vi "Power Accuracy Plot Measurement.vi"(4 "Calculated Values":refnum<vi>, 5 "Tolerance (dBm)":cluster{i32[], dbl[]}, 6 "Reset Plot? (F)":bool, 7 "Plots":T2, 8 "error in (no error)":errorcluster, 11 "Measurement Data":T1) -> (0 "error out":errorcluster)   [LabVIEW 2011]
uses:
  TypeDefs/Power Accuracy Measurement Data.ctl
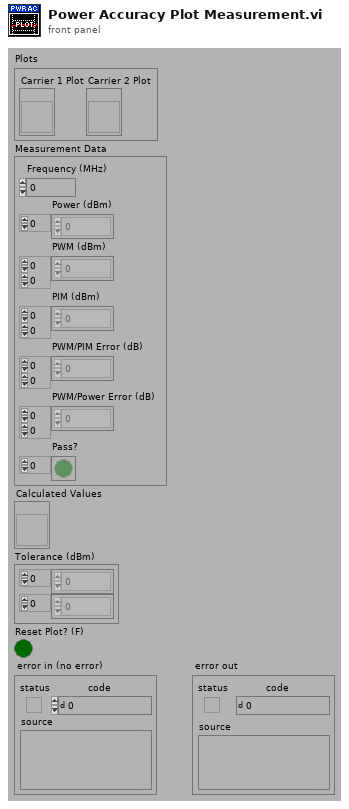
[diagram p1: front panel]
types:
  T1 = typedef "Power Accuracy Measurement Data.ctl" = cluster{"Frequency (MHz)":dbl, "Power (dBm)":i32[], "PWM (dBm)":dbl[][], "PIM (dBm)":dbl[][], "PWM/PIM Error (dB)":dbl[][], "PWM/Power Error (dB)":dbl[][], "Pass?":bool[]}
  T2 = cluster{"Carrier 1 Plot":refnum<vi>, "Carrier 2 Plot":refnum<vi>}
  T3 = cluster{"Array Constant":dbl[], "Array Constant":dbl[]}[]
  T4 = cluster{"Power (dBm)":i32[], "PWM/Power Error (dB)":dbl[]}
  T5 = cluster{"Power (dBm)":i32[], "PWM/PIM Error (dB)":dbl[]}
  T6 = cluster{"Power (dBm)":i32[], "PWM/Power Error (dB)":dbl[]}[]
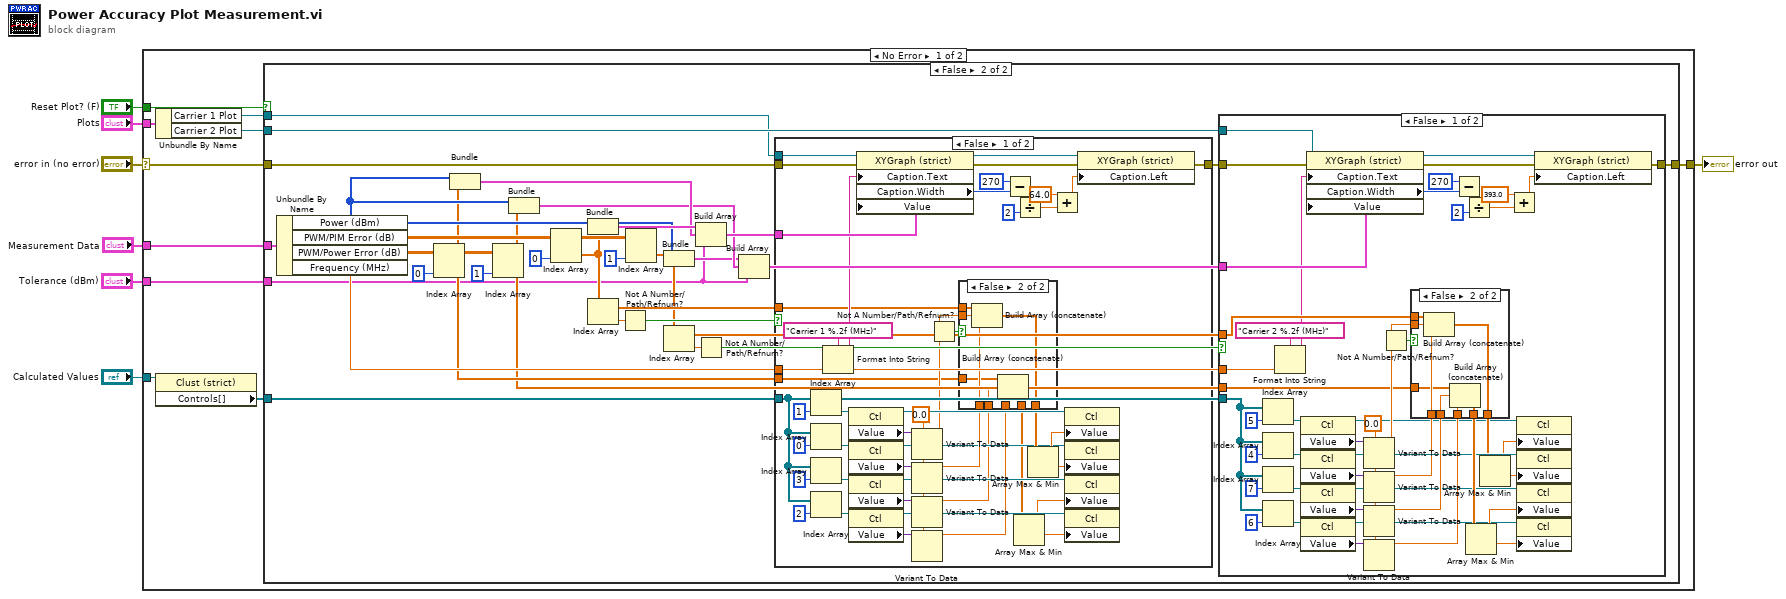
[diagram p0: block diagram]
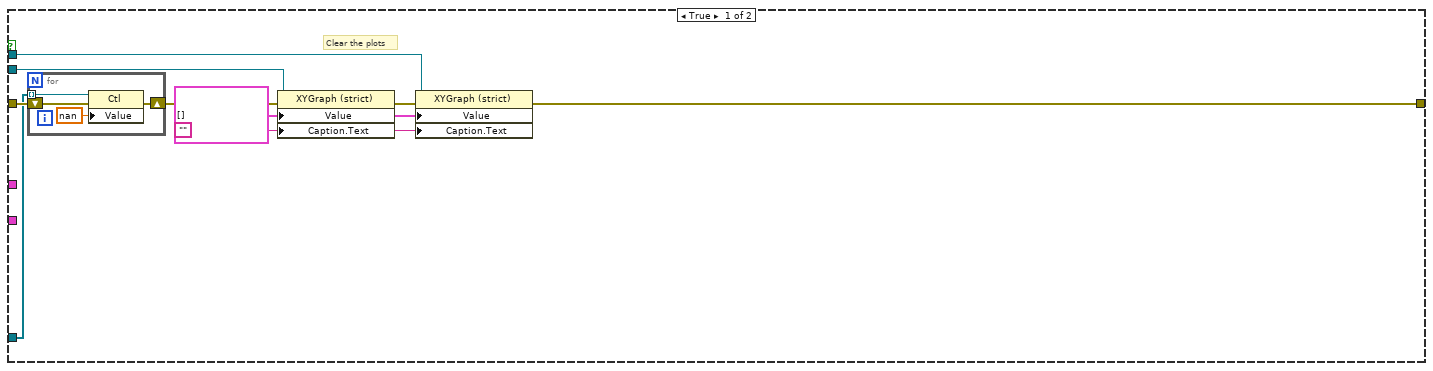
[diagram p2: hidden frame]
diagram:
  n1 = case shown="No Error" "error in (no error)" {
    selector: "error in (no error)" -> [w17 w176]
    tunnel: "Reset Plot? (F)" -> [w8 _]
    tunnel: [w9 w176] -> w6
    tunnel: "Measurement Data" -> [w16 _]
    tunnel: "Tolerance (dBm)" -> [w15 _]
    tunnel: "Plots" -> [w14 _]
    tunnel: "Calculated Values" -> [w11 _]
    frame No Error {
      n2 = Unbundle By Name(w14) -> ("Carrier 1 Plot"=w13:refnum<vi>, "Carrier 2 Plot"=w12:refnum<vi>)
      n3 = property class="Clust (strict)"(reference=w11) -> ("Controls[]"=w10:refnum<vi>[])  [unwired: 1 in, 2 out]
      n4 = case shown="False" w8 {
        tunnel: w17 -> [w26 w44]
        tunnel: w16 -> [_ w59]
        tunnel: w15 -> [_ w31]
        tunnel: w13 -> [w25 w43]
        tunnel: w12 -> [w24 w45]
        tunnel: w10 -> [w20 w49]
        tunnel: [w19 w47] -> w9
        frame True {
          w18 = ""
          w22 = T3 [] ("Value")
          # "Clear the plots"
          n5 = for {
            shift-right: [w29] -> w21
            shift-left: w26 -> [w30]
            tunnel: w20 -> [w28] mode=indexing
            n6 = property class="Ctl"(reference=w28, error in=w30, "Value"=nan) -> (error out=w29:errorcluster)  [unwired: 1 out]
          }
          n7 = property class="XYGraph (strict)"(reference=w24, error in=w21, "Value"=w22, "Caption.Text"=w18) -> (error out=w23:errorcluster)  [unwired: 1 out]
          n8 = property class="XYGraph (strict)"(reference=w25, error in=w23, "Value"=w22, "Caption.Text"=w18) -> (error out=w19:errorcluster)  [unwired: 1 out]
        }
        frame False {
          n9 = Unbundle By Name(w59) -> ("Power (dBm)"=w39:i32[], "PWM/PIM Error (dB)"=w55:dbl[][], "PWM/Power Error (dB)"=w40:dbl[][], "Frequency (MHz)"=w46:dbl)
          n10 = Index Array(array=w40, index (col)=0 ("disabled index (col)")) -> (element=w33:dbl[])  [unwired: 1 in]
          n11 = Bundle("Power (dBm)"=w39, "PWM/Power Error (dB)"=w33) -> (w38:T4)  [unwired: 1 in]
          n12 = Index Array(array=w40, index (col)=1 ("disabled index (col)")) -> (element=w32:dbl[])  [unwired: 1 in]
          n13 = Bundle("Power (dBm)"=w39, "PWM/Power Error (dB)"=w32) -> (w37:T4)  [unwired: 1 in]
          n14 = Index Array(array=w55, index (col)=0 ("disabled index (col)")) -> (element=w36:dbl[])  [unwired: 1 in]
          n15 = Bundle("Power (dBm)"=w39, "PWM/PIM Error (dB)"=w36) -> (w51:T5)  [unwired: 1 in]
          n16 = Index Array(array=w36) -> (element=w54:dbl)  [unwired: 1 in]
          n17 = Not A Number/Path/Refnum?(number/path/refnum=w54) -> (NaN/Path/Refnum?=w53:bool)
          n18 = Index Array(array=w55, index (col)=1 ("disabled index (col)")) -> (element=w35:dbl[])  [unwired: 1 in]
          n19 = Bundle("Power (dBm)"=w39, "PWM/PIM Error (dB)"=w35) -> (w34:T5)  [unwired: 1 in]
          n20 = Index Array(array=w35) -> (element=w52:dbl)  [unwired: 1 in]
          n21 = Build Array(w51, w38, w31) -> (w58:T6)
          n22 = Not A Number/Path/Refnum?(number/path/refnum=w52) -> (NaN/Path/Refnum?=w48:bool)
          n23 = Build Array(w34, w37, w31) -> (w50:T6)
          n24 = case shown="False" w53 {
            tunnel: w43 -> [w164 _]
            tunnel: [w135 w175] -> w47
            tunnel: w44 -> [w163 w175]
            tunnel: w58 -> [w162 _]
            tunnel: w49 -> [w124 _]
            tunnel: w36 -> [w122 _]
            tunnel: w46 -> [w146 _]
            tunnel: w33 -> [w121 _]
            frame False {
              w123 = 0.0
              n25 = Index Array(array=w124, index=1) -> (element=w159:refnum<vi>)
              n26 = Index Array(array=w124, index=0) -> (element=w158:refnum<vi>)
              n27 = Index Array(array=w124, index=3) -> (element=w127:refnum<vi>)
              n28 = Index Array(array=w124, index=2) -> (element=w128:refnum<vi>)
              n29 = Format Into String(format string="Carrier 1 %.2f (MHz)", w146) -> (resulting string=w145:string)  [unwired: 2 in, 1 out]
              n30 = property class="Ctl"(reference=w159) -> (reference out=w157:refnum<vi>, "Value"=w156:variant)  [unwired: 1 in, 1 out]
              n31 = property class="Ctl"(reference=w158) -> (reference out=w151:refnum<vi>, "Value"=w155:variant)  [unwired: 1 in, 1 out]
              n32 = property class="Ctl"(reference=w127) -> (reference out=w129:refnum<vi>, "Value"=w130:variant)  [unwired: 1 in, 1 out]
              n33 = property class="Ctl"(reference=w128) -> (reference out=w133:refnum<vi>, "Value"=w131:variant)  [unwired: 1 in, 1 out]
              n34 = property class="XYGraph (strict)"(reference=w164, error in=w163, "Caption.Text"=w145, "Value"=w162) -> (reference out=w136:refnum<vi>, error out=w137:errorcluster, "Caption.Width"=w138:u32)
              n35 = Variant To Data(type=w123, Variant=w156) -> (data=w148:dbl)  [unwired: 1 in, 1 out]
              n36 = Variant To Data(type=w123, Variant=w155) -> (data=w154:dbl)  [unwired: 1 in, 1 out]
              n37 = Variant To Data(type=w123, Variant=w130) -> (data=w119:dbl)  [unwired: 1 in, 1 out]
              n38 = Variant To Data(type=w123, Variant=w131) -> (data=w118:dbl)  [unwired: 1 in, 1 out]
              n39 = Not A Number/Path/Refnum?(number/path/refnum=w148) -> (NaN/Path/Refnum?=w149:bool)
              n40 = case shown="False" w149 {
                tunnel: w154 -> [_ w174]
                tunnel: [w166 w173] -> w153
                tunnel: w122 -> [w166 w172]
                tunnel: w148 -> [_ w171]
                tunnel: w121 -> [w165 w170]
                tunnel: [w165 w167] -> w120
                tunnel: w119 -> [_ w169]
                tunnel: w118 -> [_ w168]
                frame True {
                }
                frame False {
                  n41 = Build Array (concatenate)(w172, w171, w174) -> (w173:dbl[])
                  n42 = Build Array (concatenate)(w170, w169, w168) -> (w167:dbl[])
                }
              }
              n43 = Subtract(x=u32 270, y=w138) -> (x-y=w140:u32)
              n44 = Array Max & Min(array=w120) -> (max value=w132:dbl, min value=w134:dbl)  [unwired: 2 out]
              n45 = Divide(x=w140, y=u32 2) -> (x/y=w142:dbl)
              n46 = Array Max & Min(array=w153) -> (max value=w152:dbl, min value=w150:dbl)  [unwired: 2 out]
              n47 = Add(x=64.0, y=w142) -> (x+y=w144:dbl)
              n48 = property class="Ctl"(reference=w157, "Value"=w152) -> ()  [unwired: 1 in, 2 out]
              n49 = property class="Ctl"(reference=w151, "Value"=w150) -> ()  [unwired: 1 in, 2 out]
              n50 = property class="Ctl"(reference=w129, "Value"=w132) -> ()  [unwired: 1 in, 2 out]
              n51 = property class="Ctl"(reference=w133, "Value"=w134) -> ()  [unwired: 1 in, 2 out]
              n52 = property class="XYGraph (strict)"(reference=w136, error in=w137, "Caption.Left"=w144) -> (error out=w135:errorcluster)  [unwired: 1 out]
            }
            frame True {
            }
          }
          n53 = case shown="False" w48 {
            tunnel: [w95 w117] -> _
            tunnel: w47 -> [w106 w117]
            tunnel: w50 -> [w105 _]
            tunnel: w49 -> [w64 _]
            tunnel: w35 -> [w61 _]
            tunnel: w45 -> [w104 _]
            tunnel: w46 -> [w62 _]
            tunnel: w32 -> [w63 _]
            frame False {
              w90 = 0.0
              n54 = Index Array(array=w64, index=5) -> (element=w67:refnum<vi>)
              n55 = Index Array(array=w64, index=4) -> (element=w68:refnum<vi>)
              n56 = Index Array(array=w64, index=7) -> (element=w87:refnum<vi>)
              n57 = Index Array(array=w64, index=6) -> (element=w86:refnum<vi>)
              n58 = Format Into String(format string="Carrier 2 %.2f (MHz)", w62) -> (resulting string=w60:string)  [unwired: 2 in, 1 out]
              n59 = property class="Ctl"(reference=w67) -> (reference out=w69:refnum<vi>, "Value"=w70:variant)  [unwired: 1 in, 1 out]
              n60 = property class="Ctl"(reference=w68) -> (reference out=w75:refnum<vi>, "Value"=w71:variant)  [unwired: 1 in, 1 out]
              n61 = property class="Ctl"(reference=w87) -> (reference out=w85:refnum<vi>, "Value"=w84:variant)  [unwired: 1 in, 1 out]
              n62 = property class="Ctl"(reference=w86) -> (reference out=w81:refnum<vi>, "Value"=w83:variant)  [unwired: 1 in, 1 out]
              n63 = property class="XYGraph (strict)"(reference=w104, error in=w106, "Caption.Text"=w60, "Value"=w105) -> (reference out=w97:refnum<vi>, error out=w96:errorcluster, "Caption.Width"=w94:u32)
              n64 = Variant To Data(type=w90, Variant=w70) -> (data=w78:dbl)  [unwired: 1 in, 1 out]
              n65 = Variant To Data(type=w90, Variant=w71) -> (data=w72:dbl)  [unwired: 1 in, 1 out]
              n66 = Variant To Data(type=w90, Variant=w84) -> (data=w92:dbl)  [unwired: 1 in, 1 out]
              n67 = Variant To Data(type=w90, Variant=w83) -> (data=w93:dbl)  [unwired: 1 in, 1 out]
              n68 = Not A Number/Path/Refnum?(number/path/refnum=w78) -> (NaN/Path/Refnum?=w77:bool)
              n69 = case shown="False" w77 {
                tunnel: w72 -> [_ w116]
                tunnel: [w108 w115] -> w73
                tunnel: w61 -> [w108 w114]
                tunnel: w78 -> [_ w113]
                tunnel: w63 -> [w107 w112]
                tunnel: [w107 w109] -> w91
                tunnel: w92 -> [_ w111]
                tunnel: w93 -> [_ w110]
                frame True {
                }
                frame False {
                  n70 = Build Array (concatenate)(w114, w113, w116) -> (w115:dbl[])
                  n71 = Build Array (concatenate)(w112, w111, w110) -> (w109:dbl[])
                }
              }
              n72 = Subtract(x=u32 270, y=w94) -> (x-y=w102:u32)
              n73 = Divide(x=w102, y=u32 2) -> (x/y=w100:dbl)
              n74 = Array Max & Min(array=w91) -> (max value=w82:dbl, min value=w80:dbl)  [unwired: 2 out]
              n75 = Array Max & Min(array=w73) -> (max value=w74:dbl, min value=w76:dbl)  [unwired: 2 out]
              n76 = Add(x=393.0, y=w100) -> (x+y=w98:dbl)
              n77 = property class="Ctl"(reference=w69, "Value"=w74) -> ()  [unwired: 1 in, 2 out]
              n78 = property class="Ctl"(reference=w75, "Value"=w76) -> ()  [unwired: 1 in, 2 out]
              n79 = property class="Ctl"(reference=w85, "Value"=w82) -> ()  [unwired: 1 in, 2 out]
              n80 = property class="Ctl"(reference=w81, "Value"=w80) -> ()  [unwired: 1 in, 2 out]
              n81 = property class="XYGraph (strict)"(reference=w97, error in=w96, "Caption.Left"=w98) -> (error out=w95:errorcluster)  [unwired: 1 out]
            }
            frame True {
            }
          }
        }
      }
    }
    frame Error {
    }
  }
  "error out" <- w6
